vi "Control Arm Down.vi"(11 "Avoid Race Condition":bool) -> ()   [LabVIEW 2020]
uses:
  Framework/Robot Global Data.vi
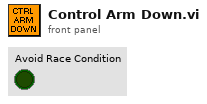
[diagram p1: front panel]
types:
  T1 = typedef "Command Status Info.ctl" = cluster{"Name":string, "Status":T2, "notifier out":T3}
  T2 = typedef "Completion Status.ctl" = enum16{"Successful", "Aborted", "Incomplete"}
  T3 = typedef "Completion Notifier.ctl" = refnum<notifier>
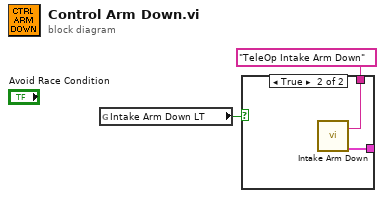
[diagram p0: block diagram]
diagram:
  n1 = global read "Robot Global Data.vi" "Intake Arm Down LT"() -> (w2:bool)
  n2 = case shown="True" w2 {
    tunnel: [_ w4] -> _
    tunnel: "TeleOp Intake Arm Down" ("Description") -> [_ w3]
    frame False {
    }
    frame True {
      n3 = call "Intake Arm Down.vi"("Description"=w3) -> ("Command Info Out"=w4:T1)  [unwired: 10 in]
    }
  }
